vi "Init Msg Input.vi"(6 "Teller":T1 {"Absolute Time" format="%<%x %.3X>T"}) -> (2 "Msg Input":refnum<class "Msg Input.lvclass">)   [LabVIEW 2020, in "jettl.lvlib" / "Start jettl Msg.lvlib" / "Start Msg Input.lvlib"]
doc: "jettl 6.14.1.98\nNathan Davis - Nathan Davis\nCopyright (c) 2026, Nathan Davis\nMIT"
uses:
  Start Msg Input.lvlib
  Msg Input/Msg Input.lvclass
  Teller Metadata/Teller Metadata.lvclass
  Start Msg Input/Start Msg Input.lvclass
  C:/git/jettl/src/jettl/jettl/Msg Input/Msg Input.lvclass
  Relation.ctl
  jettl.lvlib
  Teller.ctl
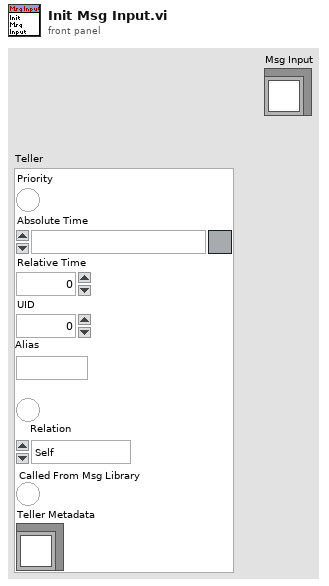
[diagram p1: front panel]
types:
  T1 = typedef "jettl.lvlib/Teller.ctl" = cluster{"Priority":bool, "Absolute Time":timestamp, "Relative Time":dbl, "UID":i32, "Alias":string, "Valid Relation":bool, "Relation":T2, "Called From Msg Library":bool, "Teller Metadata":refnum<class "Teller Metadata.lvclass">}
  T2 = typedef "jettl.lvlib/Relation.ctl" = enum16{"Self", "Parent", "Child"}
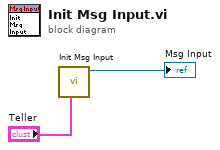
[diagram p0: block diagram]
diagram:
  n1 = call "Init Msg Input.vi"("Teller"="Teller") -> ("Start Msg Input out"=→"Msg Input":refnum<class "Start Msg Input.lvclass">)  [unwired: 10 in]
